vi "DriveDiffSetTargetSpeed.vi"(9 "Right Ft/Sec":dbl, 11 "Left Ft/Sec":dbl) -> ()   [LabVIEW 2025]
uses:
  DriveDiffGlobals.vi
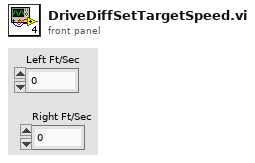
[diagram p1: front panel]
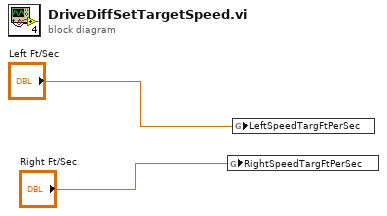
[diagram p0: block diagram]
diagram:
  n1 = global write "DriveDiffGlobals.vi" "RightSpeedTargFtPerSec"("Right Ft/Sec") -> ()
  n2 = global write "DriveDiffGlobals.vi" "LeftSpeedTargFtPerSec"("Left Ft/Sec") -> ()
